vi "Joint Points FGV.vi"(6 "Command":T1(ring), 8 "error in (no error)":errorcluster, 10 "Joint Point":cluster{"X":sgl, "Y":sgl}, 11 "name":string) -> (0 "error out":errorcluster, 2 "Joint Point":cluster{"X":sgl, "Y":sgl})   [LabVIEW 2014]
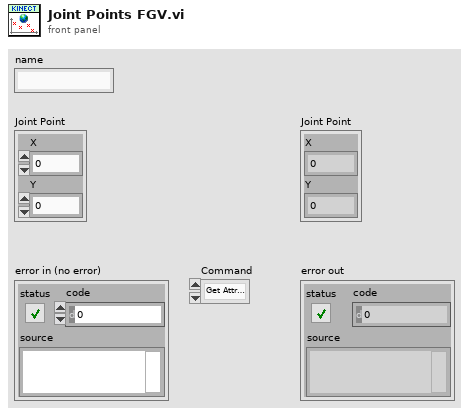
[diagram p1: front panel]
types:
  T1 = enum16{"Get Attribute", "Initialize", "Set Attribute"}
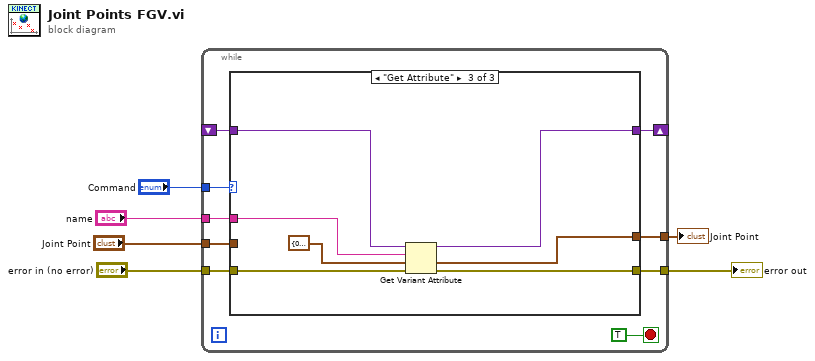
[diagram p0: block diagram]
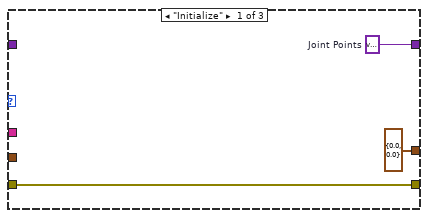
[diagram p2: hidden frame]
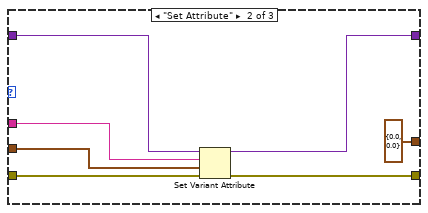
[diagram p3: hidden frame]
diagram:
  n1 = while {
    tunnel: "Command" -> [w14]
    shift-right: [w13] -> _
    shift-left: _ -> [w12]
    tunnel: "error in (no error)" -> [w11]
    tunnel: "name" -> [w10]
    tunnel: [w9] -> w3
    tunnel: "Joint Point" -> [w8]
    tunnel: [w7] -> w1
    stop <- TRUE stop-if-true
    n2 = case shown="\"Get Attribute\"" w14 {
      tunnel: [w18 w21 w28] -> w13
      tunnel: w12 -> [_ w25 w31]
      tunnel: w11 -> [w17 w24 w32]
      tunnel: w10 -> [_ w23 w30]
      tunnel: [w17 w22 w29] -> w9
      tunnel: w8 -> [_ w20 _]
      tunnel: [cluster{"X":sgl, "Y":sgl} {"X"=0.0, "Y"=0.0} ("Joint Point") cluster{"X":sgl, "Y":sgl} {"X"=0.0, "Y"=0.0} ("Joint Point") w26] -> w7
      frame "Initialize" {
        w18 = variant  # Joint Points
      }
      frame "Set Attribute" {
        n3 = Set Variant Attribute(Variant=w25, name=w23, value=w20, error in=w24) -> (Variant out=w21:variant, error out=w22:errorcluster)  [unwired: 1 out]
      }
      frame "Get Attribute" {
        n4 = Get Variant Attribute(Variant=w31, name=w30, default value (empty Variant)=cluster{"X":sgl, "Y":sgl} {"X"=0.0, "Y"=0.0} ("Joint Point"), error in=w32) -> (duplicate Variant=w28:variant, value=w26:cluster{"X":sgl, "Y":sgl}, error out=w29:errorcluster)  [unwired: 1 out]
      }
    }
  }
  "error out" <- w3
  "Joint Point" <- w1
